vi "S30c_dll F100.vi"(4 "error in":errorcluster, 6 "Index":u8, 7 "Dev Addr":u8=250) -> (0 "error out":errorcluster, 2 "Parameters 0 .. 4":u8[](array[numeric]), 3 "Parameters as cluster":T1)   [LabVIEW 2014, in "K_S30c_dll.lvlib"]
uses:
  K_S30c_dll.lvlib
  s30c.dll
panel:
  # "Function 100: Read configuration\n\nusing s30c.dll\nKeller AG für Druckmesstechnik, 29.5.08 b.v."
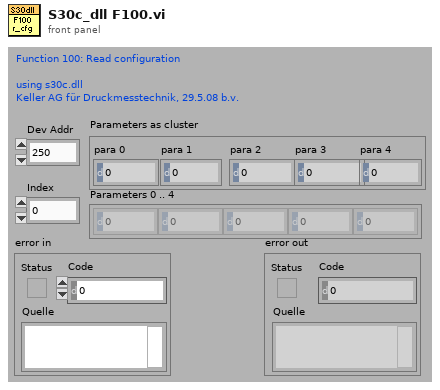
[diagram p1: front panel]
types:
  T1 = cluster{"para 0":u8, "para 1":u8, "para 2":u8, "para 3":u8, "para 4":u8}
  T2 = cluster{"Angehängtes Array[0]":u8, "Angehängtes Array[1]":u8, "Angehängtes Array[2]":u8, "Angehängtes Array[3]":u8, "Angehängtes Array[4]":u8}
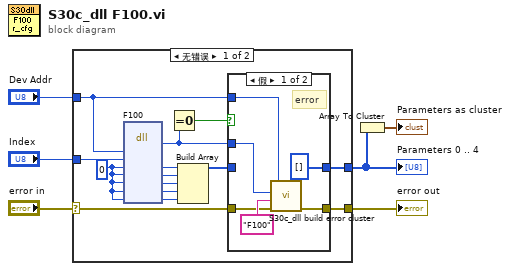
[diagram p0: block diagram]
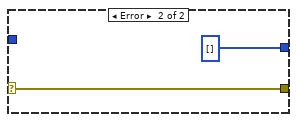
[diagram p3: hidden frame]
diagram:
  n1 = case shown="无错误" "error in" {
    selector: "error in" -> [w18 w30]
    tunnel: [w19 w30] -> w4
    tunnel: "Dev Addr" -> [w8 _]
    tunnel: "Index" -> [w15 _]
    tunnel: [w17 u8[] [] ("Angehängtes Array")] -> w3
    frame No Error {
      w16 = u8 0
      n2 = dll-call lib="PTH2Labs EworkSINOPEC北控自动相渗software2.08.5_dlls30c.dll" fn="F100"("DevAddr"=w8, "index"=w15, "Para0"=w16, "Para1"=w16, "Para2"=w16, "Para3"=w16, "Para4"=w16) -> (w9:i16, "Para0"=w14:u8, "Para1"=w13:u8, "Para2"=w12:u8, "Para3"=w11:u8, "Para4"=w10:u8)  [unwired: 5 in, 2 out]
      n3 = Equal To 0?(x=w9) -> (x = 0?=w20:bool)
      n4 = Build Array(w14, w13, w12, w11, w10) -> (w7:u8[])
      n5 = case shown="假" w20 {
        tunnel: [w26 w28] -> w19
        tunnel: w9 -> [w24 _]
        tunnel: w8 -> [w25 _]
        tunnel: w18 -> [w22 w28]
        tunnel: [u8[] [] ("Angehängtes Array") w27] -> w17
        tunnel: w7 -> [_ w27]
        frame False {
          # "error"
          n6 = call "S30c_dll build error cluster.vi"("error in"=w22, "error Text"="F100", "error code"=w24, "Dev Addr"=w25) -> ("error out"=w26:errorcluster)  [unwired: 3 in]
        }
        frame True {
        }
      }
    }
    frame Error {
    }
  }
  "error out" <- w4
  "Parameters 0 .. 4" <- w3
  n7 = Array To Cluster(array=w3) -> (cluster=→"Parameters as cluster":T2)
